vi "PH_Beckhoff_PP_Control.declare digital OutputTags.vi"() -> (0 "Digital Outputs":T2, 1 "Description":string)   [LabVIEW 2014, in "PH_Beckhoff_PP_Control.lvlib"]
uses:
  PH_Beckhoff_PP_Control.lvlib
  PH_Beckhoff/PH_Beckhoff.Digital Outputs.ctl
  PH_Beckhoff/PH_Beckhoff.lvlib
panel:
  in  "Digital Output Value":T1
  out "Right Size?":bool
  # "Let this VI run to check the size!"
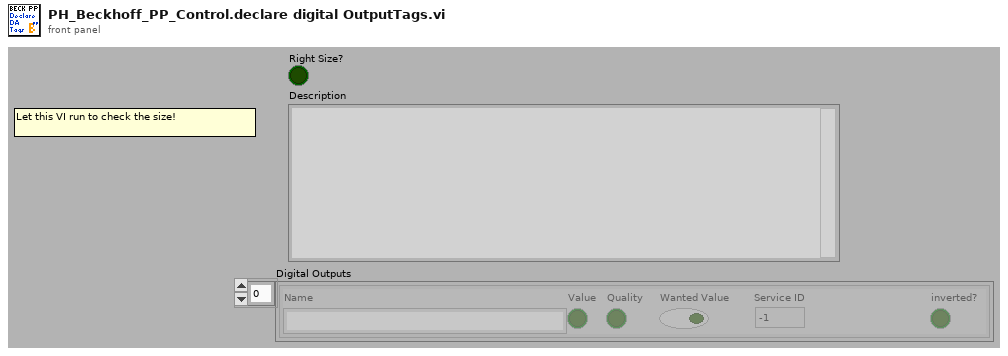
[diagram p1: front panel]
types:
  T1 = cluster{"Name":string, "Value":bool, "Quality":bool, "Wanted Value":bool, "Service ID":i32, "inverted?":bool}
  T2 = typedef "PH_Beckhoff.lvlib/PH_Beckhoff.Digital Outputs.ctl" = cluster{"Name":string, "Value":bool, "Quality":bool, "Wanted Value":bool, "Service ID":i32, "inverted?":bool}[]
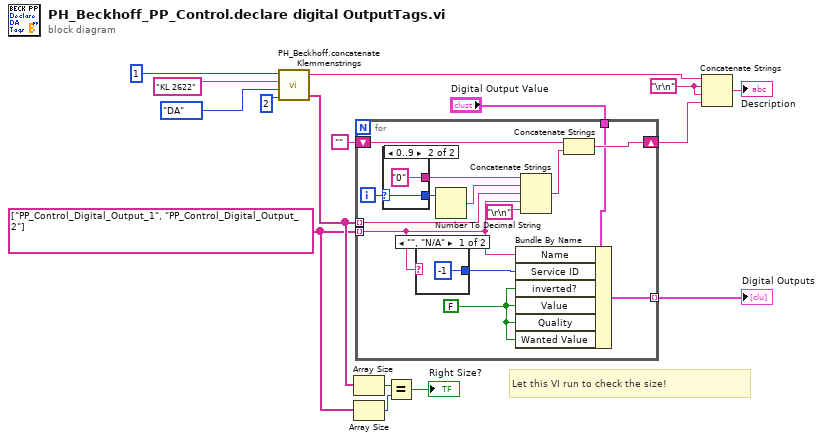
[diagram p0: block diagram]
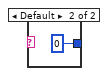
[diagram p2: hidden frame]
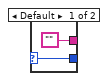
[diagram p3: hidden frame]
diagram:
  w3 = string[] ["PP_Control_Digital_Output_1", "PP_Control_Digital_Output_2"] ("appended array")
  w13 = "\r\n"
  # "Let this VI run to check the size!"
  n1 = call "PH_Beckhoff.concatenate Klemmenstrings.vi"("# of In- or Outputs"=2, "Type"=enum16{"AE", "AA", "DE", "DA"}."DA", "Klemmenname"="KL 2622", "Quantity"=1 ("size(s)")) -> ("concatenated string array"=w5:string[], "\"<Type>: <Quantity> x <Klemmenname>\""=w4:string)  [unwired: 1 out]
  n2 = Array Size(array=w5) -> (size(s)=w9:i32)
  n3 = Array Size(array=w3) -> (size(s)=w8:i32)
  n4 = for {
    tunnel: w3 -> [w20] mode=indexing
    tunnel: w5 -> [w26] mode=indexing
    shift-right: [w23] -> w14
    shift-left: "" -> [w22]
    tunnel: "Digital Output Value" -> [w21]
    tunnel: [w17] -> w1 mode=indexing
    i -> [w30]
    w18 = FALSE
    n5 = case shown="0..9" w30 {
      selector: w30 -> [w33 w36]
      tunnel: [w33 w36] -> w29
      tunnel: ["" "0"] -> w28
      frame Default {
      }
      frame 0..9 {
      }
    }
    n6 = case shown="\"\", \"N/A\"" w20 {
      tunnel: [-1 0] -> w19
      frame "", "N/A" {
      }
      frame Default {
      }
    }
    n7 = Number To Decimal String(number=w29) -> (decimal integer string=w27:string)  [unwired: 1 in]
    n8 = Bundle By Name(cluster=w21, "Name"=w20, "Service ID"=w19, "inverted?"=w18, "Value"=w18, "Quality"=w18, "Wanted Value"=w18) -> (w17:T1)
    n9 = Concatenate Strings(w28, w27, w26, w20, "\r\n") -> (w24:string)
    n10 = Concatenate Strings(w22, w24) -> (w23:string)
  }
  "Digital Outputs" <- w1
  n11 = Equal?(x=w9, y=w8) -> (x = y?=→"Right Size?":bool)
  n12 = Concatenate Strings(w4, w13, w13, w14) -> (→"Description":string)
